vi "rspvtd_Connection Notify.vi"(8 "error in":errorcluster, 11 "Data in":variant) -> (0 "error out":errorcluster, 3 "Data out":T1={"Connected?"=FALSE, "DC_UID"="", "Message Priority"=enum."Normal", "IP Address"=""})   [LabVIEW 2017, in "DS TCP Server.lvlib" / "DS TCP Server.lvclass"]
doc: "This VI converts variant data contained in the associated <b>Public API Response</b> message to its correct data type.\n---"
uses:
  DS TCP Server.lvclass
  rsp_Connection Notify.ctl
  Common VIs/DC_UID.ctl
  <vilib>/addons/_Workers/Library/Classes/Message/Priority.ctl
  <vilib>/addons/_Workers/Library/Classes/Message/Message.lvclass
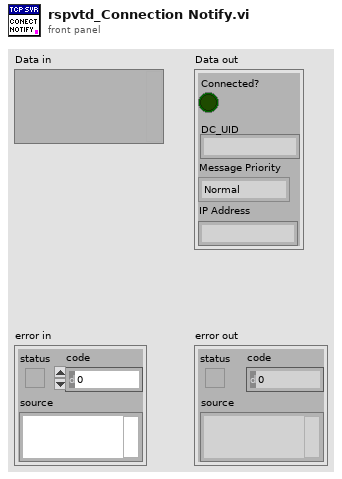
[diagram p1: front panel]
types:
  T1 = typedef "DS TCP Server.lvlib/DS TCP Server.lvclass/rsp_Connection Notify.ctl" = cluster{"Connected?":bool, "DC_UID":T2, "Message Priority":T3, "IP Address":string}
  T2 = typedef "DC_UID.ctl" = string
  T3 = typedef "Workers.lvlib/Message.lvclass/Priority.ctl" = enum16{"Low", "Normal", "High"}
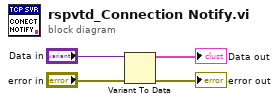
[diagram p0: block diagram]
diagram:
  n1 = Variant To Data(error in="error in", Variant="Data in") -> (data=→"Data out":T1, error out=→"error out":errorcluster)  [unwired: 1 in]
